vi "U16 array to U8 array.vi"() -> ()   [LabVIEW 2021]
panel:
  out "U8 2":u8[](array[numeric])
  out "N 2":i32
  out "time 2":u32
  out "time":u32
  out "N":i32
  out "U8":u8[](array[numeric])
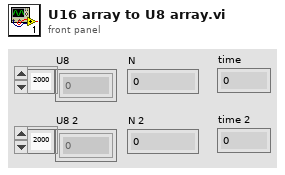
[diagram p1: front panel]
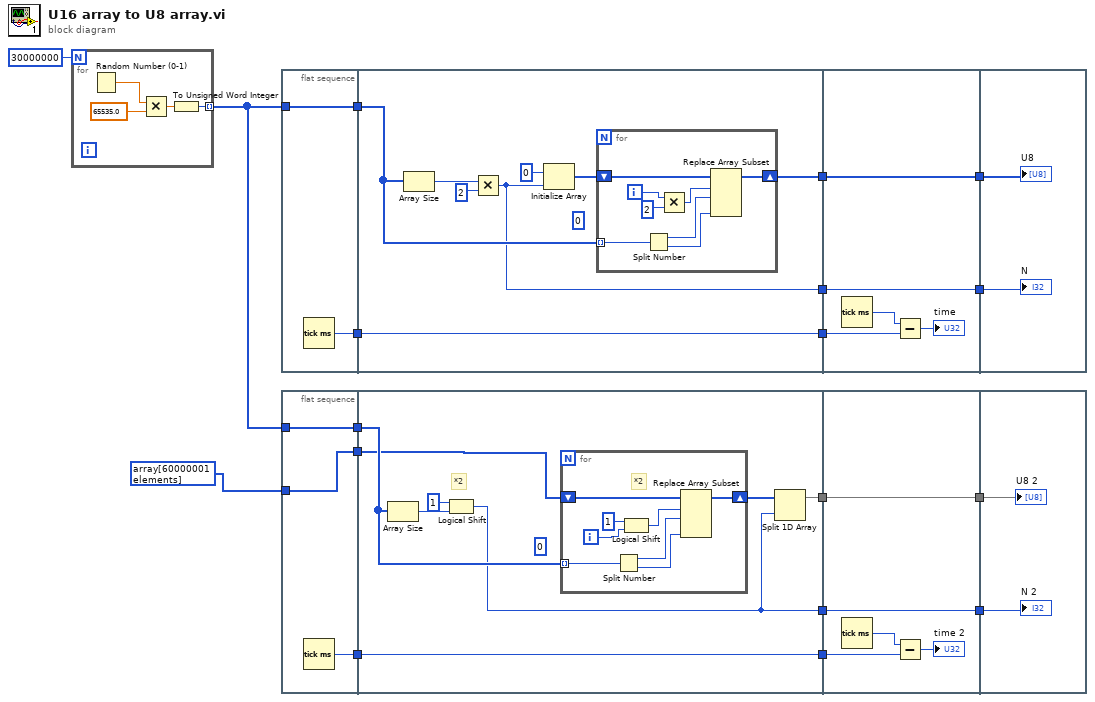
[diagram p0: block diagram]
diagram:
  n1 = for {
    N: 30000000 -> [_]
    tunnel: [w19] -> w3 mode=indexing
    n2 = Random Number (0-1)() -> (number: 0 to 1=w22:dbl)
    n3 = Multiply(x=w22, y=65535.0) -> (x*y=w20:dbl)
    n4 = To Unsigned Word Integer(number=w20) -> (unsigned 16bit integer=w19:u16)
  }
  n5 = flat-sequence {
    tunnel: w3 -> [w24]
    tunnel: [w24] -> w16
    tunnel: [w23] -> w11
    tunnel: [w25] -> w18
    tunnel: [w27] -> w17
    tunnel: w16 -> [w32]
    tunnel: [w26] -> w12
    tunnel: w11 -> [w26]
    tunnel: w18 -> [w45]
    tunnel: w17 -> [w44]
    tunnel: [w45] -> w15
    tunnel: [w44] -> w14
    tunnel: w12 -> [w42]
    tunnel: w15 -> [w47]
    tunnel: w14 -> [w46]
    frame #0 {
      n6 = Tick Count (ms)() -> (millisecond timer value=w23:u32)
    }
    frame #1 {
      (unwired) 0
      n7 = Array Size(array=w32) -> (size(s)=w31:i32)
      n8 = Multiply(x=w31, y=2) -> (x*y=w25:i32)
      n9 = Initialize Array(u8 0, w25) -> (w28:u8[])
      n10 = for {
        tunnel: w32 -> [w40] mode=indexing
        shift-right: [w38] -> w27
        shift-left: w28 -> [w39]
        i -> [w34]
        n11 = Split Number(x=w40) -> (hi(x)=w36:u8, lo(x)=w37:u8)
        n12 = Multiply(x=w34, y=2) -> (x*y=w33:i32)
        n13 = Replace Array Subset(array=w39, new element #1=w36, index #1=w33, new element #2=w37) -> (w38:u8[])  [unwired: 1 in]
      }
    }
    frame #2 {
      n14 = Tick Count (ms)() -> (millisecond timer value=w43:u32)
      n15 = Subtract(x=w43, y=w42) -> (x-y=→"time":u32)
    }
    frame #3 {
      "U8" <- w46
      "N" <- w47
    }
  }
  n16 = flat-sequence {
    tunnel: w3 -> [w50]
    tunnel: [w50] -> w10
    tunnel: [w49] -> w9
    tunnel: [w48] -> w2
    tunnel: u8[] array[60000001 elements] -> [w48]
    tunnel: [w53] -> w8
    tunnel: [w52] -> w7
    tunnel: w10 -> [w55]
    tunnel: [w58] -> w6
    tunnel: w9 -> [w58]
    tunnel: w2 -> [w51]
    tunnel: w8 -> [w71]
    tunnel: w7 -> [w70]
    tunnel: [w71] -> w5
    tunnel: [w70] -> w4
    tunnel: w6 -> [w68]
    tunnel: w5 -> [w73]
    tunnel: w4 -> [w72]
    frame #0 {
      n17 = Tick Count (ms)() -> (millisecond timer value=w49:u32)
    }
    frame #1 {
      (unwired) 0
      # "*2"
      n18 = Array Size(array=w55) -> (size(s)=w57:i32)
      n19 = Logical Shift(y=i16 1, x=w57) -> (x << y=w53:i32)
      n20 = for {
        tunnel: w55 -> [w66] mode=indexing
        shift-right: [w64] -> w54
        shift-left: w51 -> [w65]
        i -> [w60]
        # "*2"
        n21 = Split Number(x=w66) -> (hi(x)=w62:u8, lo(x)=w63:u8)
        n22 = Logical Shift(y=i16 1, x=w60) -> (x << y=w59:i32)
        n23 = Replace Array Subset(array=w65, new element #1=w62, index #1=w59, new element #2=w63) -> (w64:u8[])  [unwired: 1 in]
      }
      n24 = Split 1D Array(array=w54, index=w53) -> (first subarray=w52:u8[])  [unwired: 1 out]
    }
    frame #2 {
      n25 = Tick Count (ms)() -> (millisecond timer value=w69:u32)
      n26 = Subtract(x=w69, y=w68) -> (x-y=→"time 2":u32)
    }
    frame #3 {
      "U8 2" <- w72
      "N 2" <- w73
    }
  }
